vi "Rerouting.vi"(4 "Eye Model Cluster":T3={"X Grid"=[], "Y Grid"=[], "Za_true Surf"=[], "Iris Center"=[], "Zp_true Surf"=[], "Pinv"=[[1.0, 0.0], [0.0, 1.0]], "za_true"=5.0, "za_work"=1.0, "zp_work"=-1.0, "zp_true"=-5.0}, 5 "Trajectory Cluster":T1, 6 "PID Cluster":T6={"L1 to L4 PID Cluster"={"L1 PID Gains"={"Kp"=0.005, "Kd"=0.5, "Ki"=0.0005}, "L2 PID Gains"={"Kp"=0.01, "Kd"=1.0, "Ki"=0.005}, "L3 PID Gains"={"Kp"=0.05, "Kd"=1.0, "Ki"=0.0005}, "L4 PID Gains"={"Kp"=0.1, "Kd"=0.1, "Ki"=0.0005}}, "Stage PID Cluster"={"Stage Z PID"={"Kp"=0.0005, "Kd"=0.001, "Ki"=0.0}, "Stage Y PID"={"Kp"=0.0003, "Kd"=0.01, "Ki"=0.0}, "Stage X PID"={"Kp"=0.0003, "Kd"=0.01, "Ki"=0.0}}, "OCT Z PID Gains"={"Kp"=0.0003, "Kd"=0.0001, "Ki"=0.01}}, 7 "Offset Home 2 RCM":dbl[](array[numeric])=[0.0, 0.0, 0.0, 0.0], 8 "error in":errorcluster, 9 "Prev Index":i32, 10 "Prev Posit Cluster":T5={"Prev L1 to L4 Posit"=[-0.5319, -0.035669172703475985, -2.0566170657346783, 0.9099264705882353], "Prev Stage Posit"=[6.002553885707208, 5.996566124542428, 5.995469940427586], "Prev OCT Z Posit"=-0.0}, 11 "FPGA VI Reference In":refnum<k20>) -> (0 "error out":errorcluster, 1 "Last Index":i32, 2 "Last Posit Cluster":T4={"Last L1 to L4 Posit"=[0.0, 0.0, 0.0, 0.0], "Last Stage Posit"=[6.0, 6.0, 6.0], "Last OCT Z Posit"=0.0}, 3 "FPGA VI Reference Out":refnum<k20>)   [LabVIEW 2016]
uses:
  Global Variables.vi
  <vilib>/Platform/TimedLoop/XDataNode/wakeup.ctl
  <vilib>/Platform/TimedLoop/XDataNode/XDNodeRunTimeDep.lvlib
  <vilib>/Platform/TimedLoop/XDataNode/nitl_modes.ctl
  <vilib>/Platform/TimedLoop/XDataNode/timing_clust.ctl
  <vilib>/platform/TimedLoop/XDataNode/XDataNode.xnode
  <vilib>/Analysis/NI_AALPro.lvlib
  <vilib>/Analysis/_algsub.llb/Real Vector Norm.vi
  <vilib>/Analysis/_algsub.llb/Vector Norm Type.ctl
  <vilib>/Analysis/Matrix/Datatypes/RealMatrix.ctl
  <vilib>/Analysis/Matrix/NI_Matrix.lvlib
panel:
  out "In Servo Loop":bool
  out "Calc Finished":bool
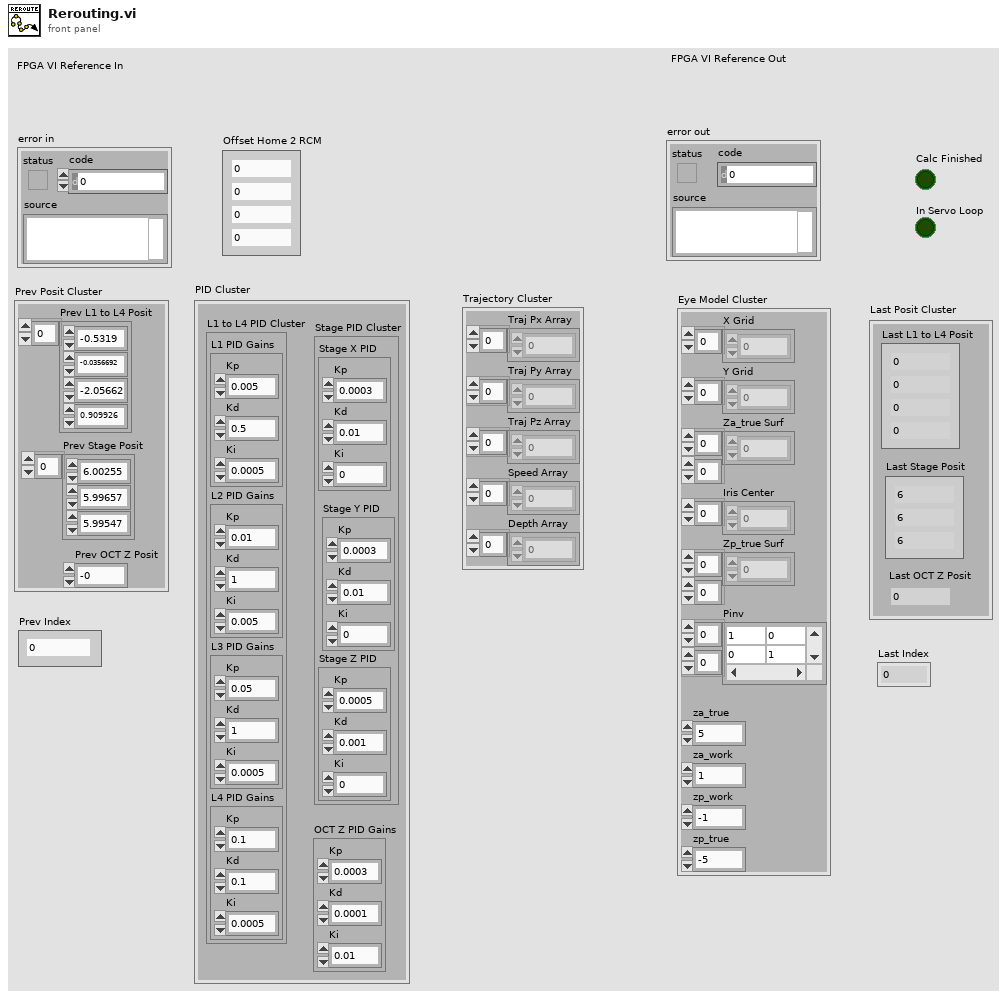
[diagram p1: front panel]
types:
  T1 = cluster{"Traj Px Array":dbl[], "Traj Py Array":dbl[], "Traj Pz Array":dbl[], "Speed Array":dbl[], "Depth Array":dbl[]}
  T2 = typedef "NI_Matrix.lvlib/RealMatrix.ctl" = dbl[][]
  T3 = cluster{"X Grid":dbl[], "Y Grid":dbl[], "Za_true Surf":dbl[][], "Iris Center":dbl[], "Zp_true Surf":dbl[][], "Pinv":T2, "za_true":dbl, "za_work":dbl, "zp_work":dbl, "zp_true":dbl}
  T4 = cluster{"Last L1 to L4 Posit":dbl[], "Last Stage Posit":dbl[], "Last OCT Z Posit":dbl}
  T5 = cluster{"Prev L1 to L4 Posit":dbl[], "Prev Stage Posit":dbl[], "Prev OCT Z Posit":dbl}
  T6 = cluster{"L1 to L4 PID Cluster":cluster{"L1 PID Gains":cluster{"Kp":dbl, "Kd":dbl, "Ki":dbl}, "L2 PID Gains":cluster{"Kp":dbl, "Kd":dbl, "Ki":dbl}, "L3 PID Gains":cluster{"Kp":dbl, "Kd":dbl, "Ki":dbl}, "L4 PID Gains":cluster{"Kp":dbl, "Kd":dbl, "Ki":dbl}}, "Stage PID Cluster":cluster{"Stage Z PID":cluster{"Kp":dbl, "Kd":dbl, "Ki":dbl}, "Stage Y PID":cluster{"Kp":dbl, "Kd":dbl, "Ki":dbl}, "Stage X PID":cluster{"Kp":dbl, "Kd":dbl, "Ki":dbl}}, "OCT Z PID Gains":cluster{"Kp":dbl, "Kd":dbl, "Ki":dbl}}
  T7 = typedef "XDNodeRunTimeDep.lvlib/timing_clust.ctl" = cluster{"Expected End [f-1]":u64, "Actual End [f-1]":u64, "Finished Late? [f-1]":bool, "Expected End [i-1]":u64, "Actual End [i-1]":u64, "Finished Late? [i-1]":bool, "Expected Start [i]":u64, "Actual Start [i]":u64, "Expected Start [f]":u64, "Actual Start [f]":u64, "Source Name":string, "Structure Name":string, "Period":i64, "Deadline":i64, "Offset":i64, "Start":i64, "Priority":i32, "Timeout":i32, "Mode":T8, "Wakeup Reason":T9, "Error":errorcluster, "Source Type":string, "Secondary Source Type":string, "Global End Time":u64, "Global Start Time":u64, "Frame Duration":u64, "Iteration Duration":u64, "Assigned CPU":i32, "I/O Scan Engine Mode":u32}
  T8 = typedef "XDNodeRunTimeDep.lvlib/nitl_modes.ctl" = enum32{"No Change", "Process missed periods, maintain original phase", "Discard missed periods, maintain original phase", "Process missed periods, ignore original phase", "Discard missed periods, ignore original phase"}
  T9 = typedef "XDNodeRunTimeDep.lvlib/wakeup.ctl" = enum32{"Normal", "Aborted", "Asynchronous wakeup", "Timing source error", "Timed loop error", "Timeout"}
  T10 = cluster{"Stop Vacuum":bool, "Vacuum Force":i8, "Max Limit [mmHg]":dbl, "Slide in":i8, "Irrigation?":bool}
  T11 = cluster{"L1 PID Gains":cluster{"Kp":dbl, "Kd":dbl, "Ki":dbl}, "L2 PID Gains":cluster{"Kp":dbl, "Kd":dbl, "Ki":dbl}, "L3 PID Gains":cluster{"Kp":dbl, "Kd":dbl, "Ki":dbl}, "L4 PID Gains":cluster{"Kp":dbl, "Kd":dbl, "Ki":dbl}}
  T12 = cluster{"Stage Z PID":cluster{"Kp":dbl, "Kd":dbl, "Ki":dbl}, "Stage Y PID":cluster{"Kp":dbl, "Kd":dbl, "Ki":dbl}, "Stage X PID":cluster{"Kp":dbl, "Kd":dbl, "Ki":dbl}}
  T13 = typedef "NI_AALPro.lvlib/Vector Norm Type.ctl" = u16
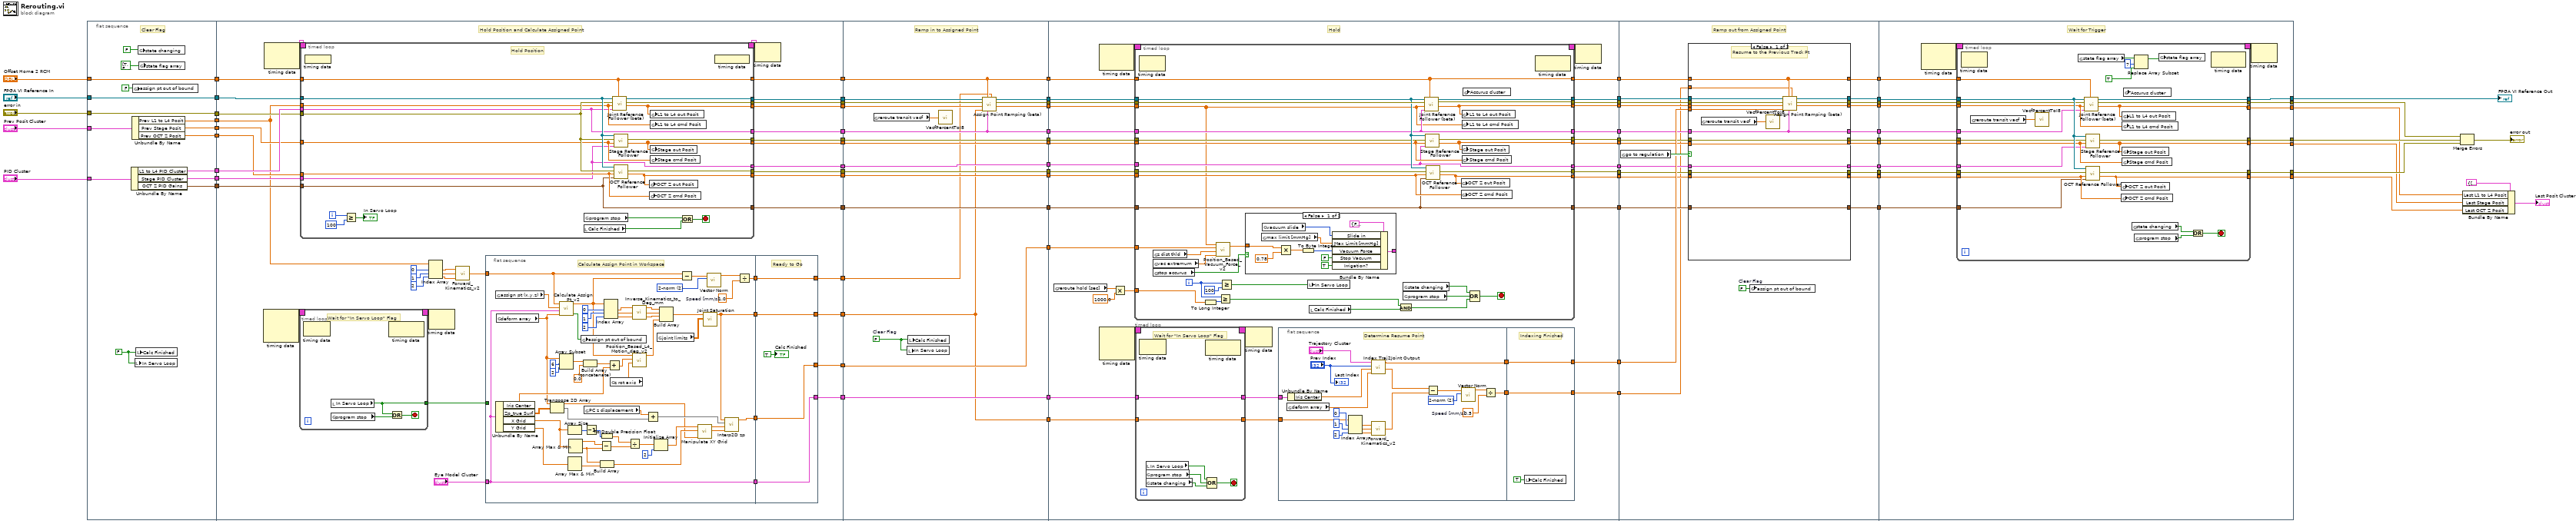
[diagram p0: block diagram]
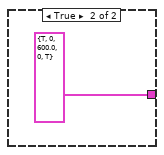
[diagram p2: hidden frame]
diagram:
  n1 = flat-sequence {
    tunnel: [w90] -> w77
    tunnel: "FPGA VI Reference In" -> [w90]
    tunnel: [w89] -> w75
    tunnel: "error in" -> [w89]
    tunnel: "Prev Posit Cluster" -> [w88]
    tunnel: "PID Cluster" -> [w87]
    tunnel: [w86] -> w73
    tunnel: [w85] -> w72
    tunnel: "Offset Home 2 RCM" -> [w84]
    tunnel: [w84] -> w70
    tunnel: [w83] -> w67
    tunnel: [w82] -> w66
    tunnel: [w81] -> w65
    tunnel: [w80] -> w64
    tunnel: w77 -> [w120]
    tunnel: w75 -> [w116]
    tunnel: w73 -> [w118]
    tunnel: w72 -> [w117]
    tunnel: w70 -> [w121]
    tunnel: w67 -> [w106]
    tunnel: w66 -> [w115]
    tunnel: w65 -> [w114]
    tunnel: w64 -> [w119]
    tunnel: [w133] -> w53
    tunnel: [w132] -> w52
    tunnel: [w131] -> w51
    tunnel: [w130] -> w50
    tunnel: [w129] -> w49
    tunnel: [w128] -> w48
    tunnel: [w127] -> w47
    tunnel: [w126] -> w46
    tunnel: [w113] -> w45
    tunnel: [w112] -> w44
    tunnel: [w111] -> w43
    tunnel: [w101] -> w8
    tunnel: [w97] -> w6
    tunnel: [w95] -> w5
    tunnel: [w93] -> w3
    tunnel: w53 -> [w236]
    tunnel: [w235] -> w42
    tunnel: w52 -> [w237]
    tunnel: [w237] -> w41
    tunnel: w51 -> [w228]
    tunnel: [w232] -> w40
    tunnel: w50 -> [w243]
    tunnel: [w243] -> w39
    tunnel: w49 -> [w242]
    tunnel: [w242] -> w38
    tunnel: w48 -> [w241]
    tunnel: [w241] -> w37
    tunnel: w47 -> [w231]
    tunnel: [w231] -> w36
    tunnel: w46 -> [w240]
    tunnel: [w240] -> w35
    tunnel: w45 -> [w234]
    tunnel: [w233] -> w34
    tunnel: w44 -> [w239]
    tunnel: [w239] -> w33
    tunnel: w43 -> [w238]
    tunnel: [w238] -> w32
    tunnel: [w229] -> w9
    tunnel: w8 -> [w229]
    tunnel: w6 -> [w225]
    tunnel: w5 -> [w227]
    tunnel: [w227] -> w4
    tunnel: w3 -> [w226]
    tunnel: [w225] -> w1
    tunnel: w42 -> [w278]
    tunnel: [w274] -> w31
    tunnel: w41 -> [w279]
    tunnel: [w265] -> w29
    tunnel: w40 -> [w276]
    tunnel: [w264] -> w27
    tunnel: w39 -> [w269]
    tunnel: [w262] -> w25
    tunnel: w38 -> [w267]
    tunnel: [w261] -> w23
    tunnel: w37 -> [w266]
    tunnel: [w259] -> w21
    tunnel: w36 -> [w275]
    tunnel: [w263] -> w19
    tunnel: w35 -> [w268]
    tunnel: [w258] -> w17
    tunnel: w34 -> [w277]
    tunnel: [w273] -> w15
    tunnel: w33 -> [w270]
    tunnel: [w260] -> w13
    tunnel: w32 -> [w271]
    tunnel: [w272] -> w11
    tunnel: w9 -> [w254]
    tunnel: [w255] -> w7
    tunnel: w4 -> [w251]
    tunnel: [w249] -> w2
    tunnel: w1 -> [w248]
    tunnel: w31 -> [w387]
    tunnel: [w382] -> w30
    tunnel: w29 -> [w388]
    tunnel: [w366] -> w28
    tunnel: w27 -> [w385]
    tunnel: [w380] -> w26
    tunnel: w25 -> [w376]
    tunnel: [w375] -> w24
    tunnel: w23 -> [w370]
    tunnel: [w369] -> w22
    tunnel: w21 -> [w368]
    tunnel: [w367] -> w20
    tunnel: w19 -> [w383]
    tunnel: [w377] -> w18
    tunnel: w17 -> [w374]
    tunnel: [w373] -> w16
    tunnel: w15 -> [w386]
    tunnel: [w381] -> w14
    tunnel: w13 -> [w371]
    tunnel: [w372] -> w12
    tunnel: w11 -> [w378]
    tunnel: [w379] -> w10
    tunnel: w7 -> [w384]
    tunnel: w2 -> [w364]
    tunnel: w30 -> [w435]
    tunnel: [w434] -> w62
    tunnel: [w433] -> w61
    tunnel: [w432] -> w60
    tunnel: w28 -> [w431]
    tunnel: w26 -> [w430]
    tunnel: w24 -> [w429]
    tunnel: w22 -> [w428]
    tunnel: w20 -> [w427]
    tunnel: w18 -> [w426]
    tunnel: w16 -> [w425]
    tunnel: [w424] -> w58
    tunnel: [w423] -> w57
    tunnel: [w422] -> w56
    tunnel: [w421] -> w54
    tunnel: w14 -> [w420]
    tunnel: w12 -> [w419]
    tunnel: w10 -> [w418]
    frame #0 {
      w79 = FALSE ("Loading Finished")
      # "Clear Flag"
      n2 = Unbundle By Name(w87) -> ("L1 to L4 PID Cluster"=w85:T11, "Stage PID Cluster"=w86:T12, "OCT Z PID Gains"=w80:cluster{"Kp":dbl, "Kd":dbl, "Ki":dbl})
      n3 = Unbundle By Name(w88) -> ("Prev L1 to L4 Posit"=w83:dbl[], "Prev Stage Posit"=w82:dbl[], "Prev OCT Z Posit"=w81:dbl)
      n4 = global write "Global Variables.vi" "assign pt out of bound"(FALSE ("assign pt out of bound")) -> ()
      n5 = local write "In Servo Loop"(w79) -> ()
      n6 = local write "Calc Finished"(w79) -> ()
      n7 = global write "Global Variables.vi" "state changing"(FALSE ("state changing")) -> ()
      n8 = global write "Global Variables.vi" "state flag array"(bool[] [TRUE, FALSE, FALSE, FALSE, FALSE, FALSE, FALSE, FALSE, FALSE] ("state flag array")) -> ()
    }
    frame #1 {
      # "Hold Position and Calculate Assigned Point"
      n9 = node-c288() -> (w123:T7)  [unwired: 3 in]
      n10 = node-c288() -> (w125:T7)  [unwired: 2 in]
      n11 = timed-loop {
        timing: w123 -> [_]
        timing-out: [_] -> w122
        tunnel: [w191] -> w99
        stop <- w193 stop-if-true
        # "Wait for \"In Servo Loop\" Flag"
        n12 = node-c288() -> ()  [unwired: 1 in, 1 out]
        n13 = global read "Global Variables.vi" "program stop"() -> (w192:bool)
        n14 = local read "In Servo Loop"() -> (w191:bool)
        n15 = node-c288() -> ()  [unwired: 1 in, 1 out]
        n16 = Or(x=w191, y=w192) -> (x .or. y?=w193:bool)
      }
      n17 = timed-loop {
        timing: w125 -> [_]
        timing-out: [_] -> w124
        tunnel: w106 -> [w213]
        tunnel: w115 -> [w211]
        tunnel: w118 -> [w201]
        tunnel: w117 -> [w202]
        tunnel: w116 -> [w215]
        tunnel: w120 -> [w216]
        tunnel: w121 -> [w208]
        tunnel: w114 -> [w209]
        tunnel: w119 -> [w203]
        tunnel: [w214] -> w131
        tunnel: [w212] -> w130
        tunnel: [w210] -> w129
        tunnel: [w208] -> w132
        tunnel: [w207] -> w133
        tunnel: [w206] -> w113
        tunnel: [w205] -> w111
        tunnel: [w204] -> w112
        tunnel: [w203] -> w128
        tunnel: [w202] -> w127
        tunnel: [w201] -> w126
        i -> [w200]
        stop <- w219 stop-if-true
        # "Hold Position"
        n18 = node-c288 ("Output Node")() -> ()  [unwired: 1 in]
        n19 = Greater Or Equal?(x=w200, y=100) -> (x >= y?=→"In Servo Loop":bool)
        n20 = local read "Calc Finished"() -> (w218:bool)
        n21 = global read "Global Variables.vi" "program stop"() -> (w217:bool)
        n22 = call "Joint Reference Follower (beta).vi"("Offset Home2RCM [deg/mm]"=w208, "PID Ctrl Cluster"=w202, "Ref Array [deg/mm]"=w213, "error in"=w215, "FPGA VI Reference In"=w216) -> ("Output Posit Array [deg/mm]"=w214:dbl[], "error out"=w206:errorcluster, "FPGA VI Reference Out"=w207:refnum<k20>)  [unwired: 4 in]
        n23 = call "Stage Reference Follower.vi"("Stage PID Cluster"=w201, "Stage cmd Posit [mm]"=w211, "error in"=w215, "FPGA VI Reference In"=w216) -> ("Stage out Posit [mm]"=w212:dbl[], "error out"=w205:errorcluster)  [unwired: 5 in, 1 out]
        n24 = call "OCT Reference Follower.vi"("OCT Z PID Gains"=w203, "OCT  Z cmd Posit [mm]"=w209, "error in"=w215, "FPGA VI Reference In"=w216) -> ("OCT  Z out Posit [mm]"=w210:dbl, "error out"=w204:errorcluster)  [unwired: 5 in, 1 out]
        n25 = global write "Global Variables.vi" "OCT Z out Posit"(w210) -> ()
        n26 = global write "Global Variables.vi" "OCT Z cmd Posit"(w209) -> ()
        n27 = global write "Global Variables.vi" "L1 to L4 out Posit"(w214) -> ()
        n28 = global write "Global Variables.vi" "L1 to L4 cmd Posit"(w213) -> ()
        n29 = global write "Global Variables.vi" "Stage out Posit"(w212) -> ()
        n30 = global write "Global Variables.vi" "Stage cmd Posit"(w211) -> ()
        n31 = Or(x=w217, y=w218) -> (x .or. y?=w219:bool)
        n32 = node-c288() -> ()  [unwired: 1 out]
      }
      n33 = Index Array(array=w106, index #1=0 ("index"), index #2=1 ("index"), index #3=2 ("index")) -> (element #1=w109:dbl, element #2=w108:dbl, element #3=w107:dbl)
      n34 = node-c288(w122) -> ()  [unwired: 1 out]
      n35 = call "Forward_Kinematics_v2.vi"("theta 3"=w107, "theta 2"=w108, "theta 1"=w109) -> ("position"=w102:dbl[])
      n36 = flat-sequence {
        tunnel: "Eye Model Cluster" -> [w162]
        tunnel: w102 -> [w153]
        tunnel: [w162] -> w100
        tunnel: w99 -> [_]
        tunnel: [w135] -> w98
        tunnel: [w154] -> w96
        tunnel: [w148] -> w94
        tunnel: [w189] -> w101
        tunnel: w100 -> [w189]
        tunnel: [w188] -> w97
        tunnel: w98 -> [w188]
        tunnel: [w186] -> w95
        tunnel: w96 -> [w186]
        tunnel: [w187] -> w93
        tunnel: w94 -> [w187]
        frame #0 {
          w149 = 1.0  # Speed [mm/s]
          w151 = T13 2 items=["1-norm"=1, "2-norm"=2, "Inf-norm"=3, "-Inf-norm"=4, "User Defined"=5] ("norm type")
          # "Calculate Assign Point in Workspace"
          n37 = global read "Global Variables.vi" "assign pt (x,y,z)"() -> (w185:dbl[])
          n38 = Unbundle By Name(w162) -> ("Iris Center"=w139:dbl[], "Zp_true Surf"=w172:dbl[][], "X Grid"=w171:dbl[], "Y Grid"=w163:dbl[])
          n39 = global read "Global Variables.vi" "deform array"() -> (w138:dbl[])
          n40 = Transpose 2D Array(2D array=w172) -> (transposed array=w157:dbl[][])
          n41 = call "Calculate Assign Pt_v2.vi"("Deform Array"=w138, "Eye Model Cluster"=w162, "Assign Pt"=w185, "Current Pt"=w153) -> ("Assign Pt OOB"=w184:bool, "Assign Pt*"=w146:dbl[])  [unwired: 6 in]
          n42 = Array Subset(array=w138, index=6, length=2) -> (w137:dbl[])
          n43 = Array Size(array=w171) -> (size(s)=w164:i32)
          n44 = Array Max & Min(array=w163) -> (min value=w167:dbl)  [unwired: 3 out]
          n45 = Array Max & Min(array=w171) -> (max value=w166:dbl, min value=w165:dbl)  [unwired: 2 out]
          n46 = global write "Global Variables.vi" "assign pt out of bound"(w184) -> ()
          n47 = Build Array (concatenate)(w137, 0.0) -> (w143:dbl[])
          n48 = global read "Global Variables.vi" "PC z displacement"() -> (w158:dbl)
          n49 = Decrement(x=w164) -> (x-1=w169:i32)
          n50 = Subtract(x=w166, y=w165) -> (x-y=w170:dbl)
          n51 = To Double Precision Float(number=w169) -> (double precision float=w168:dbl)
          n52 = Build Array(w165, w167) -> (w155:dbl[])
          n53 = Index Array(array=w146, index #1=0 ("index"), index #2=1 ("index"), index #3=2 ("index")) -> (element #1=w180:dbl, element #2=w179:dbl, element #3=w178:dbl)
          n54 = Add(x=w143, y=w139) -> (x+y=w140:dbl[])
          n55 = global read "Global Variables.vi" "z rot axis"() -> (w145:dbl)
          n56 = Divide(x=w168, y=w170) -> (x/y=w160:dbl)
          n57 = call "Inverse_Kinematics_to_Deg_mm.vi"("pz"=w178, "py"=w179, "px"=w180) -> ("L3 [mm]"=w175:dbl, "L2 [deg]"=w176:dbl, "L1 [deg]"=w177:dbl)
          n58 = call "Position_Based_L4_Motion_deg_v2.vi"("Assign z"=w145, "Iris Center"=w140, "Tip Position"=w146) -> ("L4 Motion [deg]"=w147:dbl)  [unwired: 8 in]
          n59 = Add(x=w158, y=w157) -> (x+y=w156:dbl[][])
          n60 = Initialize Array(w160, 2 ("dimension size")) -> (w159:dbl[])
          n61 = global read "Global Variables.vi" "joint limits"() -> (w134:dbl[][])
          n62 = Build Array(w177, w176, w175, w147) -> (w136:dbl[])
          n63 = Subtract(x=w153, y=w146) -> (x-y=w152:dbl[])
          n64 = call "Manipulate XY Grid.vi"("Deform Array"=w138, "XY Grid min In"=w155, "XY Quant. Fact. In"=w159) -> ("XY Grid min Out"=w173:dbl[], "XY Quant. Fact. Out"=w174:dbl[])  [unwired: 7 in]
          n65 = call "Joint Saturation.vi"("Joint Bounds [Deg/mm]"=w134, "Ref Array [Deg/mm]"=w136) -> ("Sat Ref Array [Deg/mm]"=w135:dbl[])  [unwired: 9 in]
          n66 = call-poly <vilib>:"Vector Norm.vi"("norm type"=w151, "Input Vector"=w152) -> ("norm"=w150:dbl)  [unwired: 8 in, 1 out]
          n67 = call "Interp2D zp.vi"("XY Grid min"=w173, "XY Quantization Factor"=w174, "Zp array"=w156, "Tip Position"=w135) -> ("zp"=w154:dbl)  [unwired: 7 in]
          n68 = Divide(x=w150, y=w149) -> (x/y=w148:dbl)
        }
        frame #1 {
          # "Ready to Go"
          "Calc Finished" <- TRUE ("Loading Finished")
        }
      }
      n69 = node-c288(w124) -> ()  [unwired: 1 out]
    }
    frame #2 {
      w230 = FALSE  # Clear Flag
      # "Ramp in to Assigned Point"
      n70 = global read "Global Variables.vi" "reroute transit vacf"() -> (w224:dbl)
      n71 = local write "In Servo Loop"(w230) -> ()
      n72 = local write "Calc Finished"(w230) -> ()
      n73 = call "VacfPercentToI8.vi"("vacf (0-100)"=w224) -> ()  [unwired: 1 out]
      n74 = call "Assign Point Ramping (beta).vi"("Ramp Time [sec]"=w226, "L1 to L4 PID Cluster"=w231, "Offset Home2RCM"=w237, "Destination Posit Array [mm]"=w225, "Previous Posit Array"=w228, "error in"=w234, "FPGA VI Reference In"=w236) -> ("Last L1 to L4 Posit"=w232:dbl[], "error out"=w233:errorcluster, "FPGA VI Reference Out"=w235:refnum<k20>)  [unwired: 2 in]
    }
    frame #3 {
      # "Hold"
      n75 = global read "Global Variables.vi" "reroute hold [sec]"() -> (w246:dbl)
      n76 = node-c288() -> (w281:T7)  [unwired: 2 in]
      n77 = node-c288() -> (w257:T7)  [unwired: 3 in]
      n78 = Multiply(x=w246, y=1000.0) -> (x*y=w244:dbl)
      n79 = timed-loop {
        timing: w281 -> [_]
        timing-out: [_] -> w280
        tunnel: w279 -> [w339]
        tunnel: w278 -> [w347]
        tunnel: w277 -> [w348]
        tunnel: w276 -> [w318]
        tunnel: w275 -> [w337]
        tunnel: [w346] -> w274
        tunnel: [w345] -> w273
        tunnel: [w344] -> w272
        tunnel: w271 -> [w343]
        tunnel: w270 -> [w342]
        tunnel: w269 -> [w341]
        tunnel: w268 -> [w332]
        tunnel: w267 -> [w340]
        tunnel: w266 -> [w333]
        tunnel: [w339] -> w265
        tunnel: [w338] -> w264
        tunnel: [w337] -> w263
        tunnel: [w336] -> w262
        tunnel: [w335] -> w261
        tunnel: [w334] -> w260
        tunnel: [w333] -> w259
        tunnel: [w332] -> w258
        tunnel: w251 -> [w319]
        tunnel: w244 -> [w315]
        i -> [w331]
        stop <- w324 stop-if-true
        n80 = node-c288() -> ()  [unwired: 1 in, 1 out]
        n81 = global read "Global Variables.vi" "z dist thld"() -> (w322:dbl[])
        n82 = global read "Global Variables.vi" "vac extremum"() -> (w321:dbl[])
        n83 = global read "Global Variables.vi" "stop accurus"() -> (w320:bool)
        n84 = To Long Integer(number=w315) -> (32bit integer=w316:i32)
        n85 = call "Position_Based_Vacuum_Force_v2.vi"("vac_bnd"=w321, "z_thld"=w322, "current zp"=w319, "tip position"=w318) -> ("vacf (%)"=w323:dbl)  [unwired: 7 in]
        n86 = Greater Or Equal?(x=w331, y=w316) -> (x >= y?=w328:bool)
        n87 = Greater Or Equal?(x=w331, y=100) -> (x >= y?=w330:bool)
        n88 = case shown="False" w320 {
          tunnel: [w352 T10 {"Stop Vacuum"=TRUE, "Vacuum Force"=0, "Max Limit [mmHg]"=600.0, "Slide in"=0, "Irrigation?"=TRUE} ("Accurus Ctrl Cluster")] -> _
          tunnel: w323 -> [w351 _]
          frame False {
            n89 = global read "Global Variables.vi" "max limit [mmHg]"() -> (w356:dbl)
            n90 = global read "Global Variables.vi" "vacuum slide"() -> (w357:i8)
            n91 = Multiply(x=w351, y=0.78 ("x")) -> (x*y=w354:dbl)
            n92 = To Byte Integer(number=w354) -> (8bit integer=w353:i8)
            n93 = Bundle By Name(cluster=T10 {"Stop Vacuum"=FALSE, "Vacuum Force"=0, "Max Limit [mmHg]"=0.0, "Slide in"=0, "Irrigation?"=FALSE} ("Accurus Ctrl Cluster"), "Slide in"=w357, "Max Limit [mmHg]"=w356, "Vacuum Force"=w353, "Stop Vacuum"=FALSE ("Stop Accurus"), "Irrigation?"=TRUE) -> (w352:T10)
          }
          frame True {
          }
        }
        n94 = local write "In Servo Loop"(w330) -> ()
        n95 = local read "Calc Finished"() -> (w329:bool)
        n96 = And(x=w328, y=w329) -> (x .and. y?=w327:bool)
        n97 = global read "Global Variables.vi" "state changing"() -> (w326:bool)
        n98 = global read "Global Variables.vi" "program stop"() -> (w325:bool)
        n99 = call "Joint Reference Follower (beta).vi"("Offset Home2RCM [deg/mm]"=w339, "PID Ctrl Cluster"=w337, "Ref Array [deg/mm]"=w318, "error in"=w348, "FPGA VI Reference In"=w347) -> ("Output Posit Array [deg/mm]"=w338:dbl[], "error out"=w345:errorcluster, "FPGA VI Reference Out"=w346:refnum<k20>)  [unwired: 4 in]
        n100 = call "Stage Reference Follower.vi"("Stage PID Cluster"=w332, "Stage cmd Posit [mm]"=w341, "error in"=w343, "FPGA VI Reference In"=w347) -> ("Stage out Posit [mm]"=w336:dbl[], "error out"=w344:errorcluster)  [unwired: 5 in, 1 out]
        n101 = call "OCT Reference Follower.vi"("OCT Z PID Gains"=w333, "OCT  Z cmd Posit [mm]"=w340, "error in"=w342, "FPGA VI Reference In"=w347) -> ("OCT  Z out Posit [mm]"=w335:dbl, "error out"=w334:errorcluster)  [unwired: 5 in, 1 out]
        n102 = global write "Global Variables.vi" "OCT Z out Posit"(w335) -> ()
        n103 = global write "Global Variables.vi" "OCT Z cmd Posit"(w340) -> ()
        n104 = global write "Global Variables.vi" "L1 to L4 out Posit"(w338) -> ()
        n105 = global write "Global Variables.vi" "L1 to L4 cmd Posit"(w318) -> ()
        n106 = global write "Global Variables.vi" "Stage out Posit"(w336) -> ()
        n107 = global write "Global Variables.vi" "Stage cmd Posit"(w341) -> ()
        n108 = global read "Global Variables.vi" "Accurus cluster"() -> ()  [unwired: 1 in]
        n109 = Compound Arithmetic op=OR(w326, w325, w327) -> (w324:bool)
        n110 = node-c288() -> ()  [unwired: 1 in, 1 out]
      }
      n111 = timed-loop {
        timing: w257 -> [_]
        timing-out: [_] -> w256
        tunnel: w254 -> [w310]
        tunnel: [w310] -> w253
        tunnel: w248 -> [w305]
        tunnel: [w305] -> w247
        stop <- w309 stop-if-true
        # "Wait for \"In Servo Loop\" Flag"
        n112 = node-c288() -> ()  [unwired: 1 in, 1 out]
        n113 = local read "In Servo Loop"() -> (w307:bool)
        n114 = global read "Global Variables.vi" "program stop"() -> (w306:bool)
        n115 = global read "Global Variables.vi" "state changing"() -> (w308:bool)
        n116 = node-c288() -> ()  [unwired: 1 in, 1 out]
        n117 = Compound Arithmetic op=OR(w307, w306, w308) -> (w309:bool)
      }
      n118 = node-c288(w256) -> ()  [unwired: 1 out]
      n119 = flat-sequence {
        tunnel: w253 -> [w300]
        tunnel: [w290] -> w252
        tunnel: [w292] -> w250
        tunnel: w247 -> [w286]
        tunnel: w252 -> [w303]
        tunnel: [w303] -> w255
        tunnel: [w302] -> w249
        tunnel: w250 -> [w302]
        frame #0 {
          w296 = 0.5  # Speed [mm/s]
          w298 = T13 2 items=["1-norm"=1, "2-norm"=2, "Inf-norm"=3, "-Inf-norm"=4, "User Defined"=5] ("norm type")
          # "Determine Resume Point"
          n120 = global read "Global Variables.vi" "deform array"() -> (w293:dbl[])
          n121 = Unbundle By Name(w300) -> ("Iris Center"=w294:dbl[])
          n122 = Index Array(array=w286, index #1=0 ("index"), index #2=1 ("index"), index #3=2 ("index")) -> (element #1=w285:dbl, element #2=w284:dbl, element #3=w283:dbl)
          n123 = call "Index Traj2Joint Output.vi"("Deform Array"=w293, "Pivot Pt"=w294, "Index"="Prev Index", "Trajectory Cluster"="Trajectory Cluster") -> ("Indexed Cart Posit"=w291:dbl[], "Indexed Joit Posit"=w290:dbl[])  [unwired: 6 in]
          n124 = call "Forward_Kinematics_v2.vi"("theta 3"=w283, "theta 2"=w284, "theta 1"=w285) -> ("position"=w282:dbl[])
          n125 = Subtract(x=w291, y=w282) -> (x-y=w299:dbl[])
          n126 = call-poly <vilib>:"Vector Norm.vi"("norm type"=w298, "Input Vector"=w299) -> ("norm"=w297:dbl)  [unwired: 8 in, 1 out]
          n127 = Divide(x=w297, y=w296) -> (x/y=w292:dbl)
          "Last Index" <- "Prev Index"
        }
        frame #1 {
          # "Indexing Finished"
          n128 = local write "Calc Finished"(TRUE ("Calc Finished")) -> ()
        }
      }
      n129 = node-c288(w280) -> ()  [unwired: 1 out]
    }
    frame #4 {
      w365 = FALSE  # Clear Flag
      # "Ramp out from Assigned Point"
      n130 = global read "Global Variables.vi" "go to regulation"() -> (w389:bool)
      n131 = case shown="False" w389 {
        tunnel: w388 -> [w392 w417]
        tunnel: w387 -> [w406 w416]
        tunnel: w386 -> [w405 w415]
        tunnel: w385 -> [w404 w414]
        tunnel: w384 -> [w403 _]
        tunnel: w383 -> [w398 w413]
        tunnel: [w402 w416] -> w382
        tunnel: [w401 w415] -> w381
        tunnel: [w400 w414] -> w380
        tunnel: [w399 w412] -> w379
        tunnel: w378 -> [w399 w412]
        tunnel: [w398 w413] -> w377
        tunnel: [w397 w411] -> w375
        tunnel: w376 -> [w397 w411]
        tunnel: w374 -> [w396 w410]
        tunnel: [w396 w410] -> w373
        tunnel: [w395 w409] -> w372
        tunnel: w371 -> [w395 w409]
        tunnel: w370 -> [w394 w408]
        tunnel: [w394 w408] -> w369
        tunnel: [w393 w407] -> w367
        tunnel: w368 -> [w393 w407]
        tunnel: [w392 w417] -> w366
        tunnel: w364 -> [w391 _]
        frame False {
          # "Resume to the Previous Track Pt"
          n132 = global read "Global Variables.vi" "reroute transit vacf"() -> (w390:dbl)
          n133 = call "VacfPercentToI8.vi"("vacf (0-100)"=w390) -> ()  [unwired: 1 out]
          n134 = call "Assign Point Ramping (beta).vi"("Ramp Time [sec]"=w391, "L1 to L4 PID Cluster"=w398, "Offset Home2RCM"=w392, "Destination Posit Array [mm]"=w403, "Previous Posit Array"=w404, "error in"=w405, "FPGA VI Reference In"=w406) -> ("Last L1 to L4 Posit"=w400:dbl[], "error out"=w401:errorcluster, "FPGA VI Reference Out"=w402:refnum<k20>)  [unwired: 2 in]
        }
        frame True {
          # "Bypass if \"go to regulation\" bit is True"
        }
      }
      n135 = global write "Global Variables.vi" "assign pt out of bound"(w365) -> ()
    }
    frame #5 {
      # "Wait for Trigger"
      n136 = node-c288() -> (w437:T7)  [unwired: 2 in]
      n137 = timed-loop {
        timing: w437 -> [_]
        timing-out: [_] -> w436
        tunnel: w435 -> [w456]
        tunnel: w420 -> [w455]
        tunnel: [w454] -> w433
        tunnel: [w453] -> w434
        tunnel: [w452] -> w432
        tunnel: w431 -> [w451]
        tunnel: w430 -> [w450]
        tunnel: w429 -> [w449]
        tunnel: w428 -> [w448]
        tunnel: w427 -> [w447]
        tunnel: w426 -> [w446]
        tunnel: w425 -> [w445]
        tunnel: [w444] -> w424
        tunnel: [w443] -> w423
        tunnel: [w442] -> w422
        tunnel: [w441] -> w421
        tunnel: w419 -> [w440]
        tunnel: w418 -> [w439]
        stop <- w463 stop-if-true
        n138 = node-c288() -> ()  [unwired: 1 in, 1 out]
        n139 = global read "Global Variables.vi" "reroute transit vacf"() -> (w438:dbl)
        n140 = call "VacfPercentToI8.vi"("vacf (0-100)"=w438) -> ()  [unwired: 1 out]
        n141 = global read "Global Variables.vi" "state flag array"() -> (w460:bool[])
        n142 = call "Joint Reference Follower (beta).vi"("Offset Home2RCM [deg/mm]"=w451, "PID Ctrl Cluster"=w446, "Ref Array [deg/mm]"=w450, "error in"=w455, "FPGA VI Reference In"=w456) -> ("Output Posit Array [deg/mm]"=w444:dbl[], "error out"=w454:errorcluster, "FPGA VI Reference Out"=w441:refnum<k20>)  [unwired: 4 in]
        n143 = call "Stage Reference Follower.vi"("Stage PID Cluster"=w445, "Stage cmd Posit [mm]"=w449, "error in"=w439, "FPGA VI Reference In"=w456) -> ("Stage out Posit [mm]"=w443:dbl[], "error out"=w453:errorcluster)  [unwired: 5 in, 1 out]
        n144 = call "OCT Reference Follower.vi"("OCT Z PID Gains"=w447, "OCT  Z cmd Posit [mm]"=w448, "error in"=w440, "FPGA VI Reference In"=w456) -> ("OCT  Z out Posit [mm]"=w442:dbl, "error out"=w452:errorcluster)  [unwired: 5 in, 1 out]
        n145 = global write "Global Variables.vi" "OCT Z out Posit"(w442) -> ()
        n146 = global write "Global Variables.vi" "OCT Z cmd Posit"(w448) -> ()
        n147 = global write "Global Variables.vi" "L1 to L4 out Posit"(w444) -> ()
        n148 = global write "Global Variables.vi" "L1 to L4 cmd Posit"(w450) -> ()
        n149 = global write "Global Variables.vi" "Stage out Posit"(w443) -> ()
        n150 = global write "Global Variables.vi" "Stage cmd Posit"(w449) -> ()
        n151 = global read "Global Variables.vi" "Accurus cluster"() -> ()  [unwired: 1 in]
        n152 = global read "Global Variables.vi" "state changing"() -> (w462:bool)
        n153 = Replace Array Subset(array=w460, new element=TRUE ("new element/subarray"), index=7) -> (w459:bool[])
        n154 = global read "Global Variables.vi" "program stop"() -> (w461:bool)
        n155 = global write "Global Variables.vi" "state flag array"(w459) -> ()
        n156 = Or(x=w462, y=w461) -> (x .or. y?=w463:bool)
        n157 = node-c288() -> ()  [unwired: 1 in, 1 out]
      }
      n158 = node-c288(w436) -> ()  [unwired: 1 out]
    }
  }
  n159 = Merge Errors(w61, w62, w60) -> (→"error out":errorcluster)
  n160 = Bundle By Name(cluster=T4 {"Last L1 to L4 Posit"=[0.0, 0.0, 0.0, 0.0], "Last Stage Posit"=[6.0, 6.0, 6.0], "Last OCT Z Posit"=0.0} ("Last Posit Cluster 2"), "Last L1 to L4 Posit"=w58, "Last Stage Posit"=w57, "Last OCT Z Posit"=w56) -> (→"Last Posit Cluster":T4)
  "FPGA VI Reference Out" <- w54
